vi "TreeMap V1 to V2.vi"(8 "error in (no error)":errorcluster, 11 "V1":T1) -> (0 "error out":errorcluster, 3 "V2":T3)   [LabVIEW 2020, in "Blue Tree Map OpenSource.lvlib"]
uses:
  Blue Tree Map OpenSource.lvlib
  Typedefs/Tree Map Handle.ctl
  Typedefs/Tree Map.ctl
  Typedefs/Tree Map Data.ctl
  Typedefs/Tree Node Data.ctl
  Typedefs/Attribute Map.ctl
  Typedefs/TreeMap V1.ctl
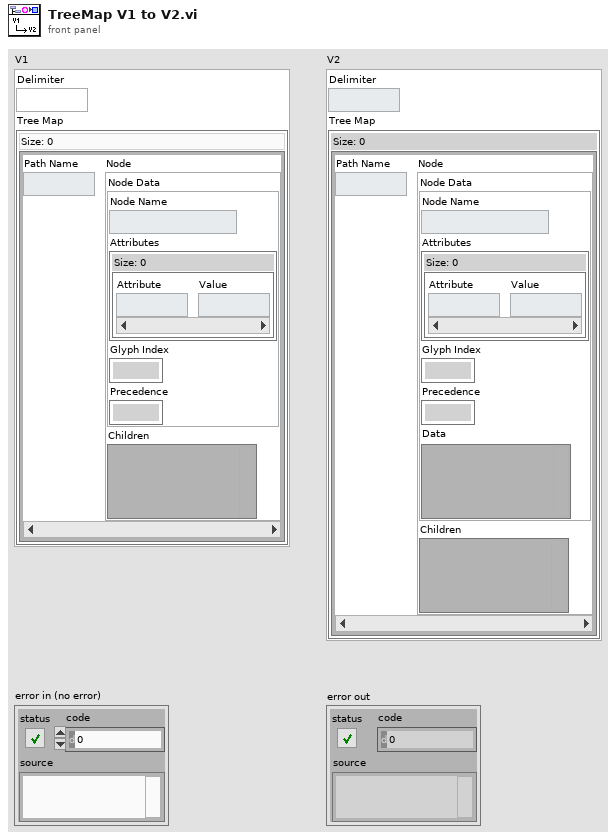
[diagram p1: front panel]
types:
  T1 = typedef "Blue Tree Map OpenSource.lvlib/TreeMap V1.ctl" = cluster{"Delimiter":string, "Tree Map":map{string, cluster{"Node Data":cluster{"Node Name":string, "Attributes":T2, "Glyph Index":i32, "Precedence":i32}, "Children":variant}}}
  T2 = typedef "Blue Tree Map OpenSource.lvlib/Attribute Map.ctl" = map{string, string}
  T3 = typedef "Blue Tree Map OpenSource.lvlib/Tree Map Handle.ctl" = cluster{"Delimiter":string, "Tree Map":T4}
  T4 = typedef "Blue Tree Map OpenSource.lvlib/Tree Map.ctl" = map{string, T5}
  T5 = typedef "Blue Tree Map OpenSource.lvlib/Tree Map Data.ctl" = cluster{"Node Data":T6, "Children":variant}
  T6 = typedef "Blue Tree Map OpenSource.lvlib/Tree Node Data.ctl" = cluster{"Node Name":string, "Attributes":T2, "Glyph Index":i32, "Precedence":i32, "Data":variant}
  T7 = map{string, cluster{"Node Data":cluster{"Node Name":string, "Attributes":T2, "Glyph Index":i32, "Precedence":i32}, "Children":variant}}
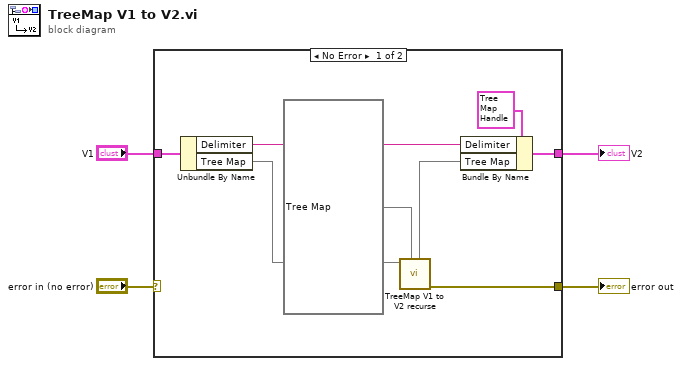
[diagram p0: block diagram]
diagram:
  n1 = case shown="No Error" "error in (no error)" {
    selector: "error in (no error)" -> [_ w13]
    tunnel: "V1" -> [w12 _]
    tunnel: [w6 _] -> w3
    tunnel: [w5 w13] -> w2
    frame No Error {
      n2 = Unbundle By Name(w12) -> ("Delimiter"=w9:string, "Tree Map"=w11:T7)
      n3 = call "TreeMap V1 to V2 recurse.vi"("V2 Map in"=T4 {}, "V1"=w11) -> ("error out"=w5:errorcluster, "V2 Map out"=w8:T4)  [unwired: 8 in]
      n4 = Bundle By Name(cluster=T3 {"Delimiter"="", "Tree Map"={}} ("V2"), "Delimiter"=w9, "Tree Map"=w8) -> (w6:T3)
    }
    frame Error {
    }
  }
  "V2" <- w3
  "error out" <- w2
